vi "gamma_correction_float.vi"(9 "i32_ar_first_and_last_pixel":i32[](array[numeric]), 10 "u8_pxar_dist":dbl[](array[numeric])) -> (3 "i16_normalized unwrapped array":dbl[](array[numeric]))   [LabVIEW 2011]
uses:
  global_vars.vi
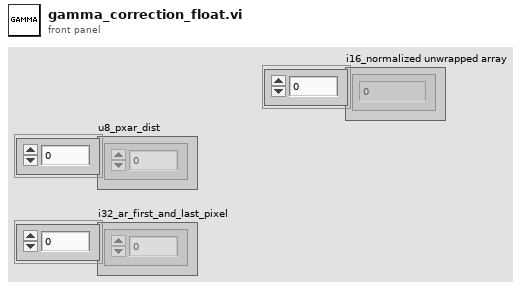
[diagram p1: front panel]
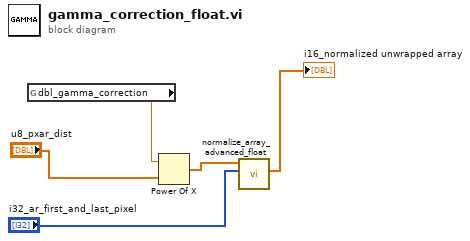
[diagram p0: block diagram]
diagram:
  n1 = global read "global_vars.vi" "dbl_gamma_correction"() -> (w1:dbl)
  n2 = Power Of X(1:"u8_pxar_dist", 2:w1) -> (0:w5:dbl[])
  n3 = call "normalize_array_advanced_float.vi"("i32_ar_first_and_last_pixel"="i32_ar_first_and_last_pixel", "unwrapped array"=w5) -> ("i16_normalized unwrapped array"=→"i16_normalized unwrapped array":dbl[])  [unwired: 5 in, 4 out]
